vi "Unicode UTF16 Change Byte Order.vi"(6 "Change BO?":bool=TRUE, 8 "error in (no error)":errorcluster, 9 "UTF-16 String In":string="…\u000b…\u000b…\u000b") -> (0 "error out":errorcluster, 1 "UTF-16 String Out":string)   [LabVIEW 2011]
doc: "Converts the UTF-16LE to UTF-16BE and vice versa."
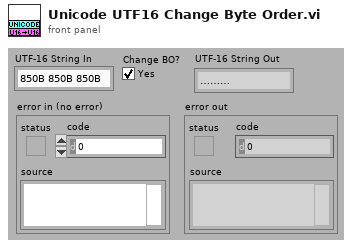
[diagram p1: front panel]
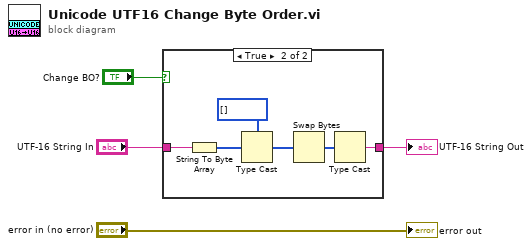
[diagram p0: block diagram]
diagram:
  n1 = case shown="True" "Change BO?" {
    tunnel: "UTF-16 String In" -> [w5 w9]
    tunnel: [w5 w6] -> w2
    frame False {
    }
    frame True {
      n2 = String To Byte Array(string=w9) -> (unsigned byte array=w11:u8[])
      n3 = Type Cast(type=u16[] [] ("[UTF-16]"), x=w11) -> (*(type *) &x=w8:u16[])
      n4 = Swap Bytes(anything=w8) -> (byte swapped=w7:u16[])
      n5 = Type Cast(x=w7) -> (*(type *) &x=w6:string)  [unwired: 1 in]
    }
  }
  "UTF-16 String Out" <- w2
  "error out" <- "error in (no error)"
